vi "CANopen.vi"() -> ()   [LabVIEW 2016]
uses:
  Ctrl/CAN_Info.ctl
  Ctrl/CAN_FrameInfo.ctl
  BusStatistics/TLIBCANBusStatistics_Ctrl.ctl
  SubVIs/MessageInfo.ctl
  Ctrl/CAN_BaudInfo.ctl
  <vilib>/Platform/TimedLoop/XDataNode/timing_clust.ctl
  <vilib>/Platform/TimedLoop/XDataNode/nitl_modes.ctl
  <vilib>/Platform/TimedLoop/XDataNode/wakeup.ctl
  <vilib>/Platform/TimedLoop/XDataNode/XDataNode.xnode
  <vilib>/Platform/TimedLoop/XDataNode/XDNodeRunTimeDep.lvlib
panel:
  in  "清除总线统计":bool
  in  "使能统计功能":bool
  out "收发总数":i32
  in  "停止":bool
  in  "配置选项卡":enum32{"APP", "CAN", "DBC", "LOG"}(tab)
  in  "APP配置":T1={"应用程序名"="APP", "CAN使用通道数"=1, "LIN使用通道数"=0} {"LIN使用通道数" max=5; "CAN使用通道数" max=5}
  out "连接状态：":bool
  in  "CAN配置":T2={"硬件类型"=3, "硬件子类型"=5, "ABaudrateKbps"=500.0, "AListenOnly"=enum."Normal", "Int120Ohm"=enum."Disable", "EnableChannel"=enum."Enable", "AHwChannel"=0, "AAppChannel"=0} {"AAppChannel" items=["CHN1", "CHN2", "CHN3", "CHN4", "CHN5", "CHN6", "CHN7", "CHN8", "CHN9", "CHN10", "CHN11", "CHN12", "CHN13", "CHN14", "CHN15", "CHN16", "CHN17", "CHN18", "CHN19", "CHN20", "CHN21", "CHN22", "CHN23", "CHN24", "CHN25", "CHN26", "CHN27", "CHN28", "CHN29", "CHN30", "CHN31", "CHN32"]; "AHwChannel" items=["CHN1", "CHN2", "CHN3", "CHN4", "CHN5", "CHN6", "CHN7", "CHN8", "CHN9", "CHN10", "CHN11", "CHN12", "CHN13", "CHN14", "CHN15", "CHN16", "CHN17", "CHN18", "CHN19", "CHN20", "CHN21", "CHN22", "CHN23", "CHN24", "CHN25", "CHN26", "CHN27", "CHN28", "CHN29", "CHN30", "CHN31", "CHN32"]; "硬件子类型" items=["BUS_UNKNOWN_TYPE", "TSCAN_PRO_4", "TSCAN_LITE_2", "TSCANMini", "TSLinMini", "TSCANFDmini", "TSCAN_LIN_IO_2", "TSCAN_LITE_2", "TSCANLIN", "TSCAN_FD_Mini_1"]; "硬件类型" items=["BUS_UNKNOWN_TYPE", "TS_TCP_DEVICE", "XL_USB_DEVICE", "TS_USB_DEVICE", "PEAK_USB_DEVICE", "KVASER_USB_DEVICE", "ZLG_USB_DEVICE", "ICS_USB_DEVICE", "TS_TC1005_DEVICE"]}
  in  "StartCAN":bool
  out "CAN状态":bool
  in  "路径":path
  in  "加载dbc":bool
  in  "SupportedChannelsBased0":string
  out "out AId":u32
  in  "Blf文件路径":path=path "D:/LabviewWorkSpace/海卓项目资料/SFCV FCURig 文件夹/BottomLevel/TS_CANDrive/Test_blf/UserBlf.blf"
  in  "开启blf记录":bool
  out "TextDisplay":string
  in  "接收选项卡":enum32{"CAN", "CANopen", "DBC"}(tab)
  out "CAN数据列表":string[][](table)
  out "接收到的原始报文：":string
  out "CORecSDOData":u32 caption="接收到的数据为" format="0x%04x"
  in  "接收子索引":u8 caption="子索引" format="0x%02x"
  in  "接收索引":u16 caption="索引" format="0x%04x"
  in  "接收从站号":u8 caption="从站号" max=127
  in  "CANopenText":string
  out "当前时间":timestamp format="%<当前时间：%Y/%m/%d  %H:%M:%S>T"
  in  "消息周期":sgl=10.0
  in  "发送选项卡":enum32{"CAN", "CANopen", "DBC"}(tab)
  in  "循环周期：":u32=10 format="%d ms"
  in  "循环发送":bool
  in  "ADLC":u8=8 caption="长度：" max=64
  in  "AIsRemote":enum16{"数据帧", "远程帧"}(ring)
  in  "AIsExt":enum16{"标准帧", "扩展帧"}(ring)
  in  "AID":u32=1234 caption="ID" max=536870911 format="0x%x"
  in  "ADataArray":u8[](array[numeric])=[0, 0, 0, 0, 0, 0, 0, 0] caption="数据0x：" format="%02x"
  in  "发送通道":i32(ring) items=["CHN1", "CHN2", "CHN3", "CHN4", "CHN5", "CHN6", "CHN7", "CHN8", "CHN9", "CHN10", "CHN11", "CHN12", "CHN13", "CHN14", "CHN15", "CHN16", "CHN17", "CHN18", "CHN19", "CHN20", "CHN21", "CHN22", "CHN23", "CHN24", "CHN25", "CHN26", "CHN27", "CHN28", "CHN29", "CHN30", "CHN31", "CHN32"]
  in  "CAN发送按钮":bool
  in  "COSDOdataW":i64 caption="写入数据:" min=-32768 max=32767
  in  "写入数据类型:":T3(ring)
  out "CANopen报文预览：":string
  out "COSDOdataS":u32 caption="SDO数据" format="0x%04x"
  in  "子索引：":u8 format="0x%02x"
  in  "索引：":u16 format="0x%04x"
  in  "操作：":enum16{"SDO快速读取请求", "SDO快速写入请求"}(ring)
  in  "从站号：":u8 max=127
  in  "CANopen发送":bool
  out "tsapp_delete_cyclic_msg_can":i32
  in  "AAppChannel":i32(ring) items=["CHN1", "CHN2", "CHN3", "CHN4", "CHN5", "CHN6", "CHN7", "CHN8", "CHN9", "CHN10", "CHN11", "CHN12", "CHN13", "CHN14", "CHN15", "CHN16", "CHN17", "CHN18", "CHN19", "CHN20", "CHN21", "CHN22", "CHN23", "CHN24", "CHN25", "CHN26", "CHN27", "CHN28", "CHN29", "CHN30", "CHN31", "CHN32"]
  in  "删除周期消息":bool
  in  "周期消息":T4 {"ADLC" max=64; "AID" max=536870911}
  in  "添加周期发送消息":bool
  out "tsapp_add_cyclic_msg_can":i32
  out "接收的数据":T5[](array[typedef])
  in  "查询内容":u16(ring) items=["获取网络名称"=0, "获取dbc文件名"=1, "获取协议类型，0=CAN、1=J1939"=2, "获取信号表数量"=10, "获取CAN报文表数量"=11, "获取CANFD报文表数量"=12, "获取CANJ1939报文表数量"=13, "获取节点表数量"=14, "获取环境变量表数量"=15, "获取取值表数量"=16, "获取信号表中第idx信号所在的报文标识符"=20, "获取信号表中第idx信号值类型"=21, "获取信号表中第idx信号是否是Motorola"=22, "获取信号表中第idx信号所带的取值表在取值表列表中的索引"=23, "获取信号表中第idx信号Mux类型"=24, "获取信号表中第idx信号作为multiplexor的值"=25, "获取信号表中第idx信号在报文中的起始位"=26, "获取信号表中第idx信号的信号长度"=27, "获取信号表中第idx信号放大因子"=28, "获取信号表中第idx信号偏移量"=29, "获取信号表中第idx信号初始值"=30, "获取信号表中第idx信号最小值"=31, "获取信号表中第idx信号最大值"=32, "获取信号表中第idx信号名称"=33, "获取信号表中第idx信号单位"=34, "获取信号表中第idx信号注释"=35, "获取信号表中第idx信号所在的报文在报文表中的索引"=36, "获取信号表中第idx信号所在的报文的类型"=37, "获取信号表中第idx信号全部属性"=38, "获取CAN报文表中第idx报文类型"=40, "获取CAN报文表中第idx报文数据长度"=41, "获取CAN报文表中第idx报文标识符"=42, "获取CAN报文表中第idx报文周期"=43, "获取CAN报文表中第idx报文名称"=44, "获取CAN报文表中第idx报文注释"=45, "获取CAN报文表中第idx报文对应的发送节点的索引"=46, "获取CAN报文表中第idx报文拥有的信号数量"=47, "获取CAN报文表中第idx报文中第subidx信号在信号表中的索引"=48, "获取CAN报文表中第idx报文全部属性"=49, "获取CANFD报文表中第idx报文属性"=60, "获取CANFD报文表中第idx报文数据长度"=61, "获取CANFD报文表中第idx报文标识符"=62, "获取CANFD报文表中第idx报文周期"=63, "获取CANFD报文表中第idx报文名称"=64, "获取CANFD报文表中第idx报文注释"=65, "获取CANFD报文表中第idx报文对应的发送节点的索引"=66, "获取CANFD报文表中第idx报文拥有的信号数量"=67, "获取CANFD报文表中第idx报文中第subidx信号在信号表中的索引"=68, "获取CANFD报文表中第idx报文BRS"=69, "获取CANFD报文表中第idx报文全部属性"=70, "获取J1939报文表中第idx报文类型"=80, "获取J1939报文表中第idx报文数据长度"=81, "获取J1939报文表中第idx报文标识符"=82, "获取J1939报文表中第idx报文周期"=83, "获取J1939报文表中第idx报文名称"=84, "获取J1939报文表中第idx报文注释"=85, "获取J1939报文表中第idx报文对应的发送节点的索引"=86, "获取J1939报文表中第idx报文拥有的信号数量"=87, "获取J1939报文表中第idx报文中第subidx信号在信号表中的索引"=88, "获取CAN报文表中第idx报文全部属性"=89, "获取节点表中第idx节点地址"=100, "获取节点表中第idx节点名称"=101, "获取取值表中第idx取值表所包含的值数量"=140, "获取取值表中第idx取值表名称"=141, "获取取值表中第idx取值表中第subidx的值"=142, "获取取值表中第idx取值表全部属性"=143]
  in  "查询dbc":bool
  out "TLIBCANBusStatistics_Ctrl":T6
  out "错误输出":errorcluster
  in  "发送数据帧信息":T4={"AID"=1234, "AIsExt"=enum."STD", "AIsRemote"=enum."Data", "ADLC"=5, "ADataArray"=[0, 0, 10, 96, 8, 8]} {"ADLC" max=64; "AID" max=536870911}
  # "win32目前没有dbc属性获取，\n需要.net方式"
  # "接收"
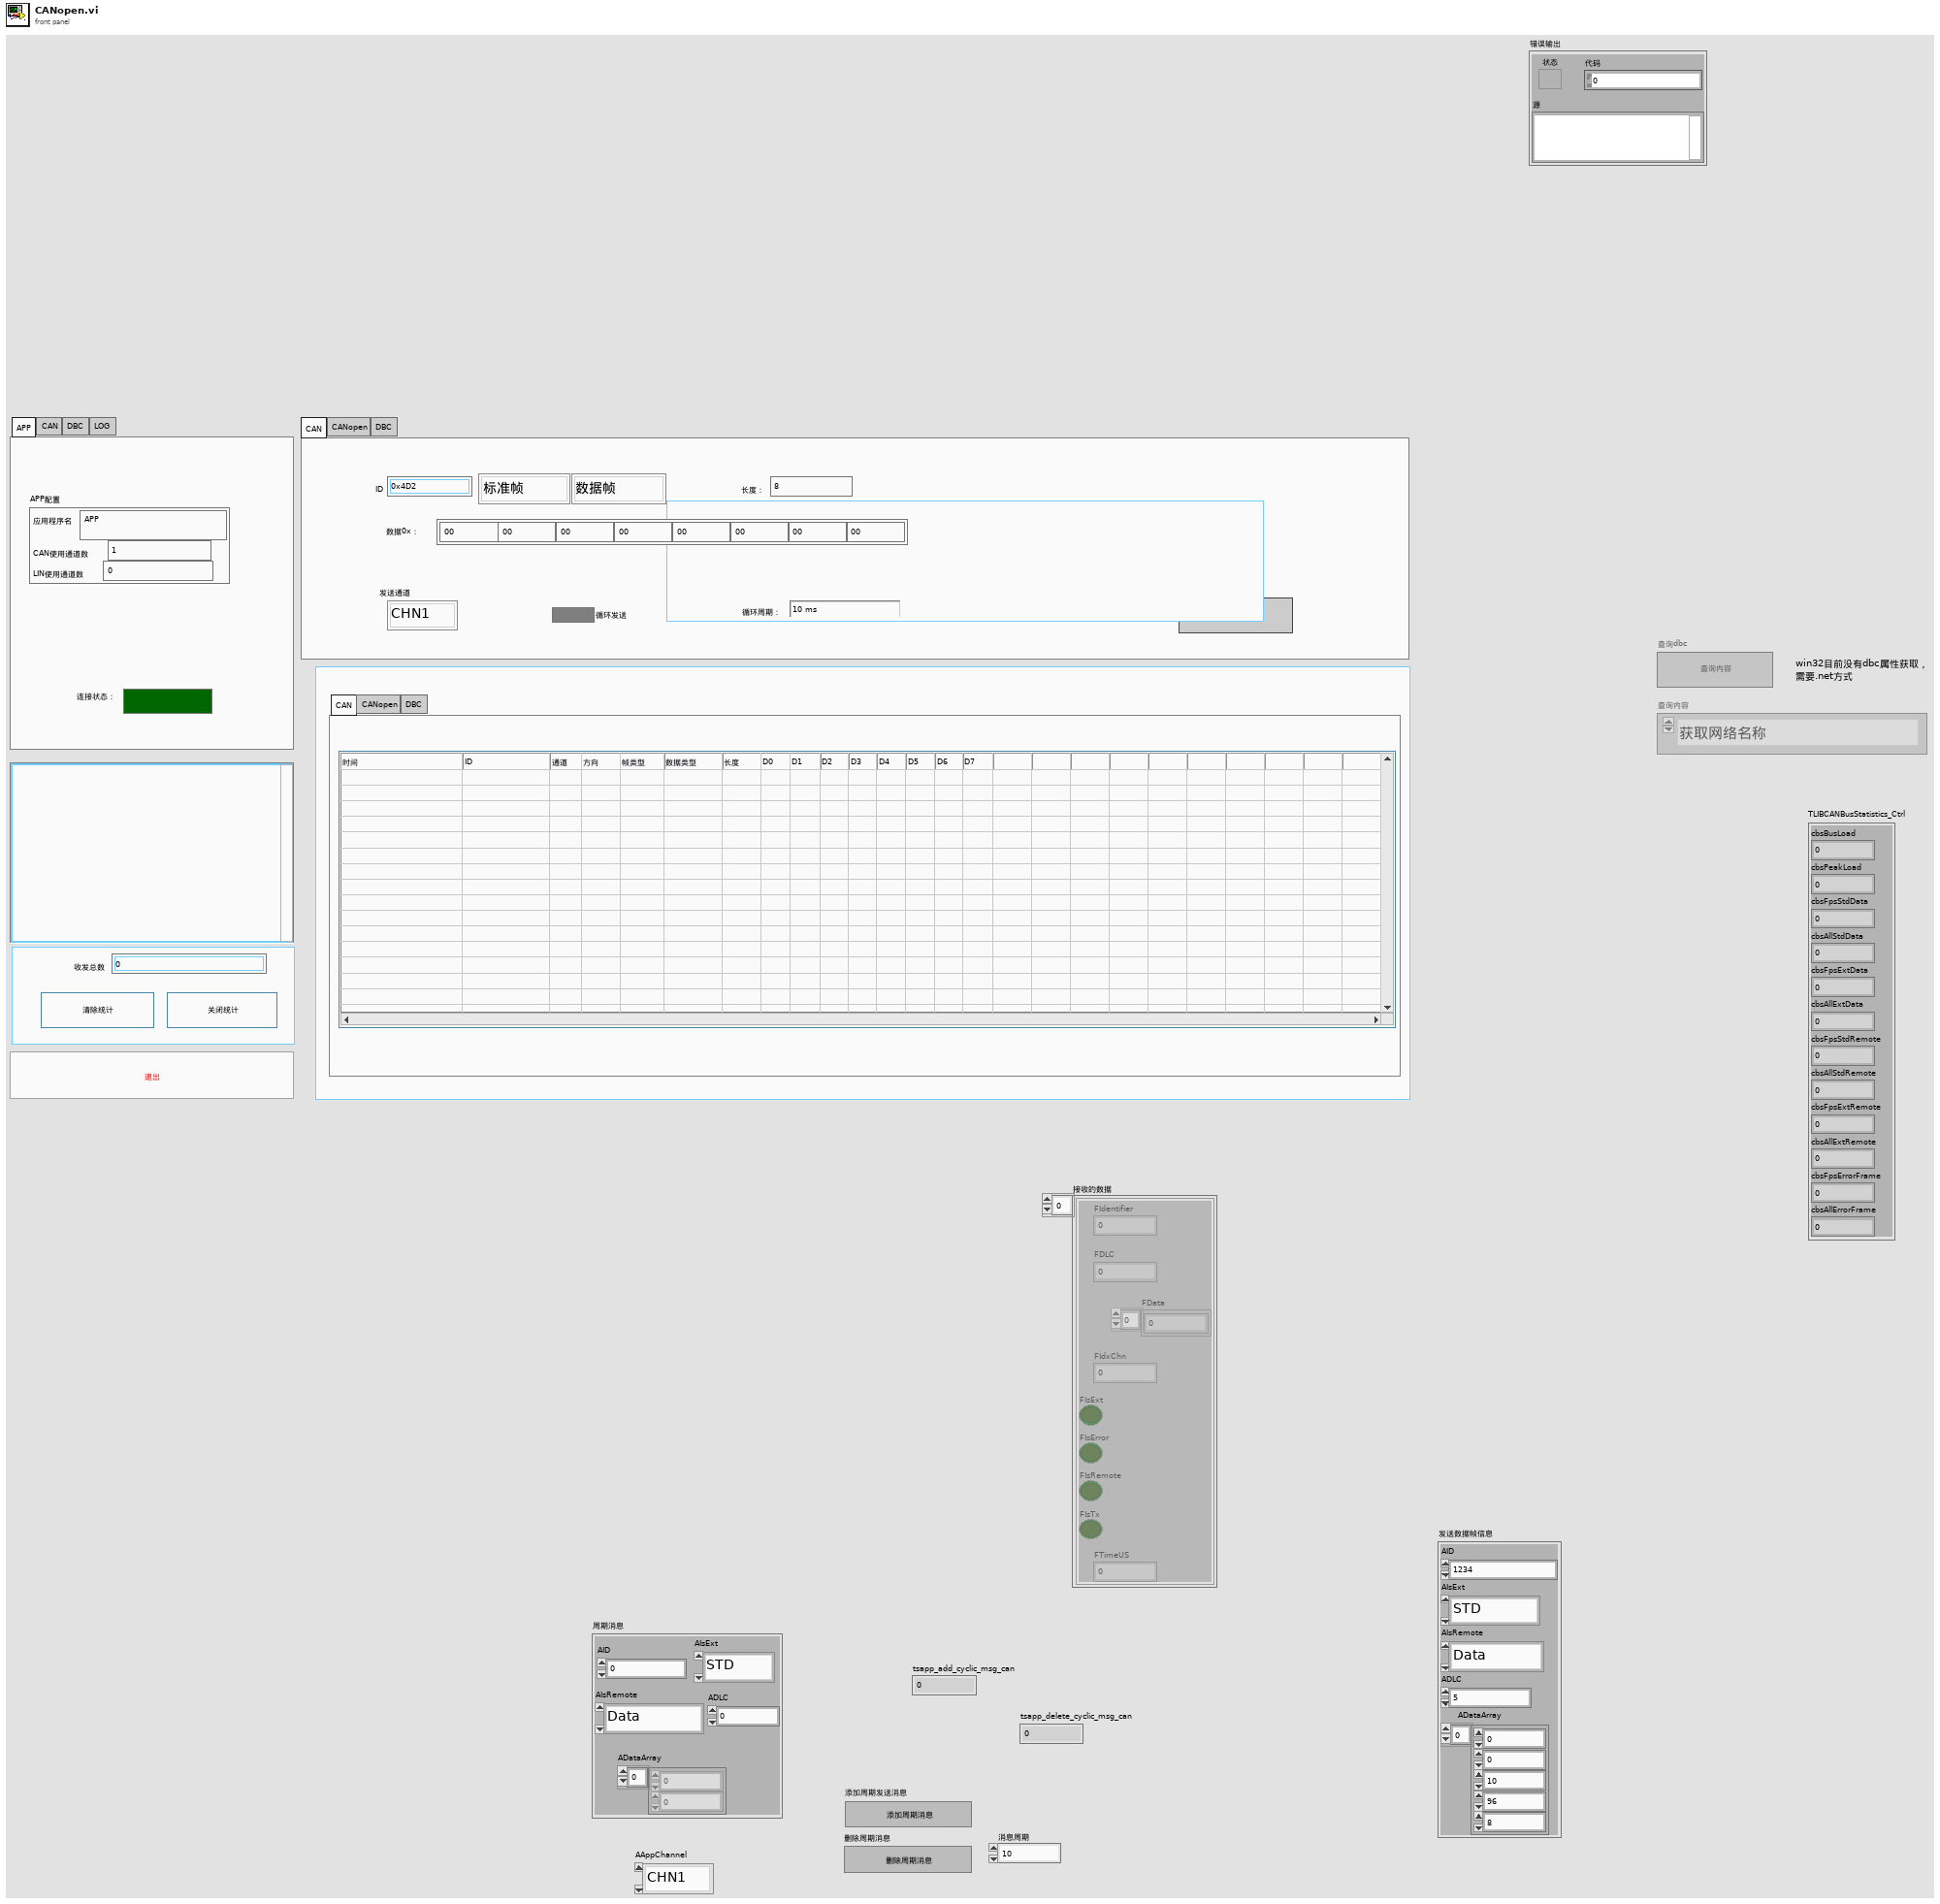
[diagram p1: front panel]
types:
  T1 = typedef "CAN_Info.ctl" = cluster{"应用程序名":string, "CAN使用通道数":u8, "LIN使用通道数":u8}
  T2 = typedef "CAN_BaudInfo.ctl" = cluster{"硬件类型":i32, "硬件子类型":i32, "ABaudrateKbps":sgl, "AListenOnly":enum16{"Normal", "ListenOnly"}, "Int120Ohm":enum16{"Disable", "Enable"}, "EnableChannel":enum16{"Disable", "Enable"}, "AHwChannel":i32, "AAppChannel":i32}
  T3 = enum16{"int8", "uint8", "int16", "uint16", "int32", "uint32"}
  T4 = typedef "CAN_FrameInfo.ctl" = cluster{"AID":u32, "AIsExt":enum16{"STD", "EXT"}, "AIsRemote":enum16{"Data", "Remote"}, "ADLC":u8, "ADataArray":u8[]}
  T5 = typedef "MessageInfo.ctl" = cluster{"FIdentifier":i32, "FDLC":u8, "FData":u8[], "FIdxChn":u8, "FIsExt":bool, "FIsError":bool, "FIsRemote":bool, "FIsTx":bool, "FTimeUS":u64}
  T6 = typedef "TLIBCANBusStatistics_Ctrl.ctl" = cluster{"cbsBusLoad":dbl, "cbsPeakLoad":dbl, "cbsFpsStdData":dbl, "cbsAllStdData":dbl, "cbsFpsExtData":dbl, "cbsAllExtData":dbl, "cbsFpsStdRemote":dbl, "cbsAllStdRemote":dbl, "cbsFpsExtRemote":dbl, "cbsAllExtRemote":dbl, "cbsFpsErrorFrame":dbl, "cbsAllErrorFrame":dbl}
  T7 = typedef "XDNodeRunTimeDep.lvlib/timing_clust.ctl" = cluster{"Expected End [f-1]":u64, "Actual End [f-1]":u64, "Finished Late? [f-1]":bool, "Expected End [i-1]":u64, "Actual End [i-1]":u64, "Finished Late? [i-1]":bool, "Expected Start [i]":u64, "Actual Start [i]":u64, "Expected Start [f]":u64, "Actual Start [f]":u64, "Source Name":string, "Structure Name":string, "Period":i64, "Deadline":i64, "Offset":i64, "Start":i64, "Priority":i32, "Timeout":i32, "Mode":T8, "Wakeup Reason":T9, "Error":errorcluster, "Source Type":string, "Secondary Source Type":string, "Global End Time":u64, "Global Start Time":u64, "Frame Duration":u64, "Iteration Duration":u64, "Assigned CPU":i32, "I/O Scan Engine Mode":u32}
  T8 = typedef "XDNodeRunTimeDep.lvlib/nitl_modes.ctl" = enum32{"No Change", "Process missed periods, maintain original phase", "Discard missed periods, maintain original phase", "Process missed periods, ignore original phase", "Discard missed periods, ignore original phase"}
  T9 = typedef "XDNodeRunTimeDep.lvlib/wakeup.ctl" = enum32{"Normal", "Aborted", "Asynchronous wakeup", "Timing source error", "Timed loop error", "Timeout"}
  T10 = enum16{"CHAN1", "CHAN2", "CHAN3", "CHAN4", "CHAN5", "CHAN6", "CHAN7", "CHAN8", "CHAN9", "CHAN10", "CHAN11", "CHAN12", "CHAN13", "CHAN14", "CHAN15", "CHAN16"}
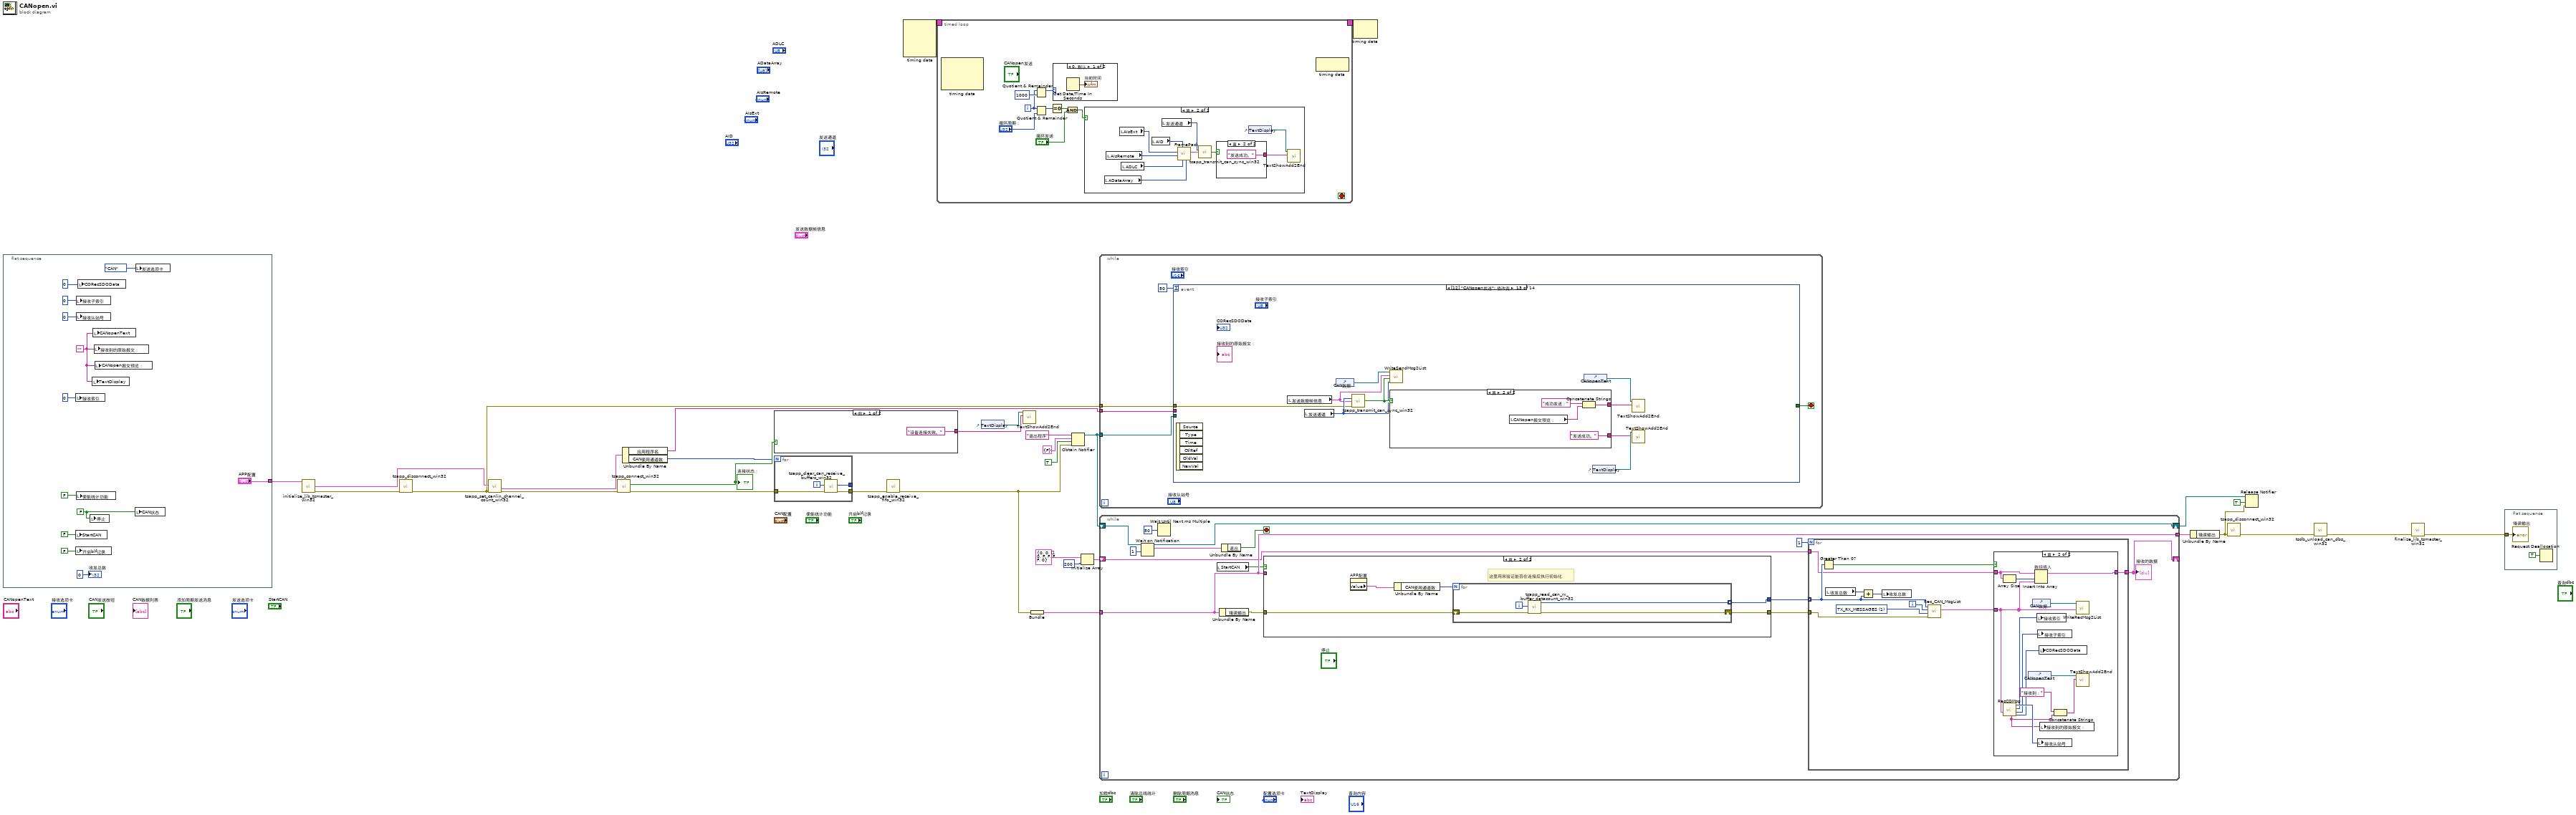
[diagram p0: block diagram]
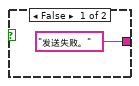
[diagram p3: hidden frame]
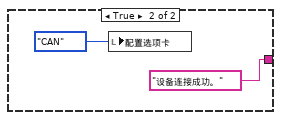
[diagram p5: hidden frame]
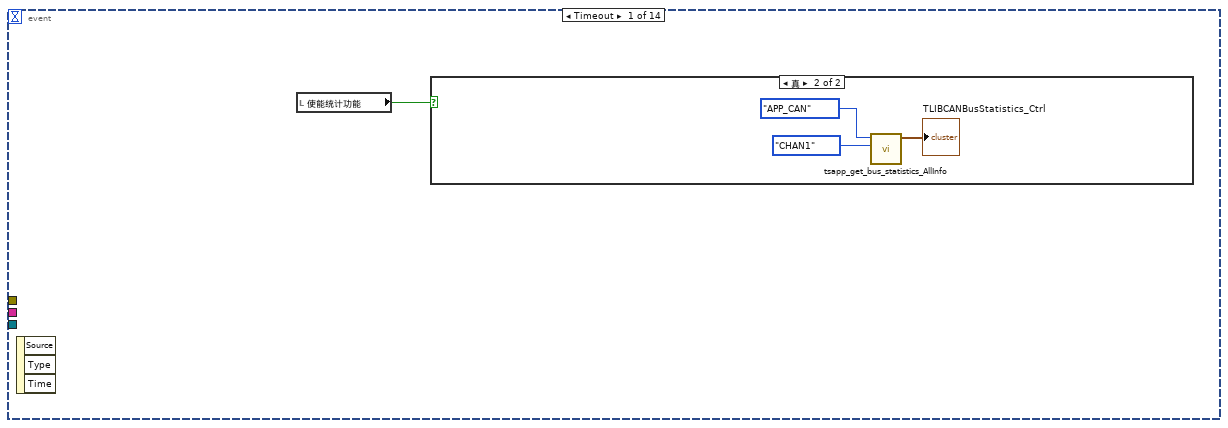
[diagram p6: hidden frame]
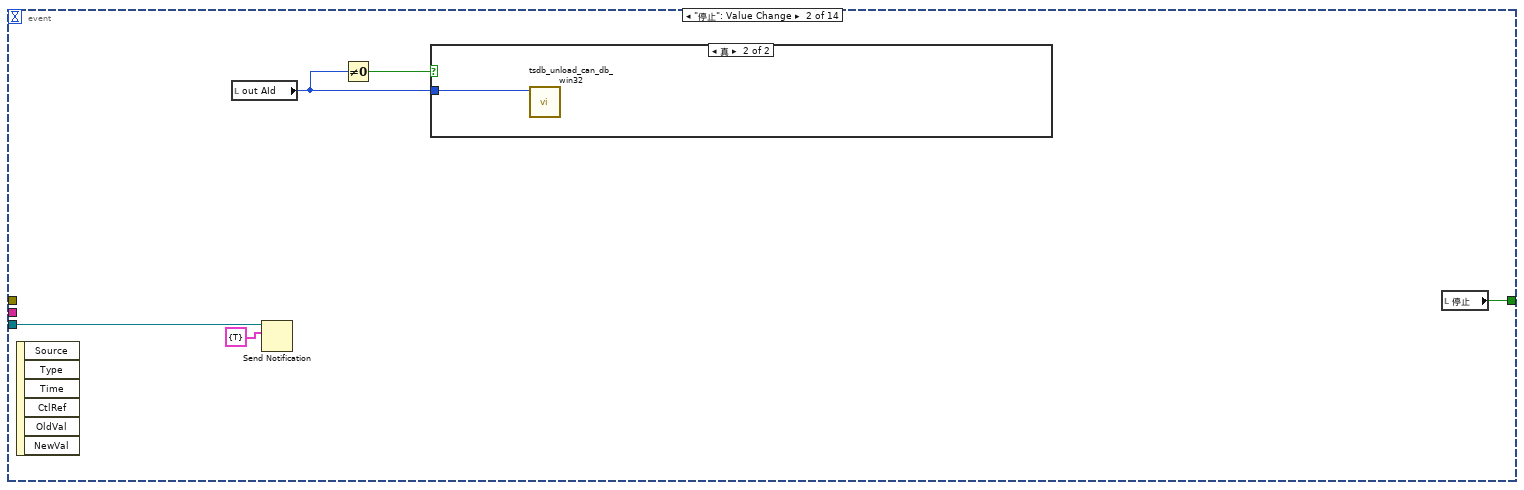
[diagram p8: hidden frame]
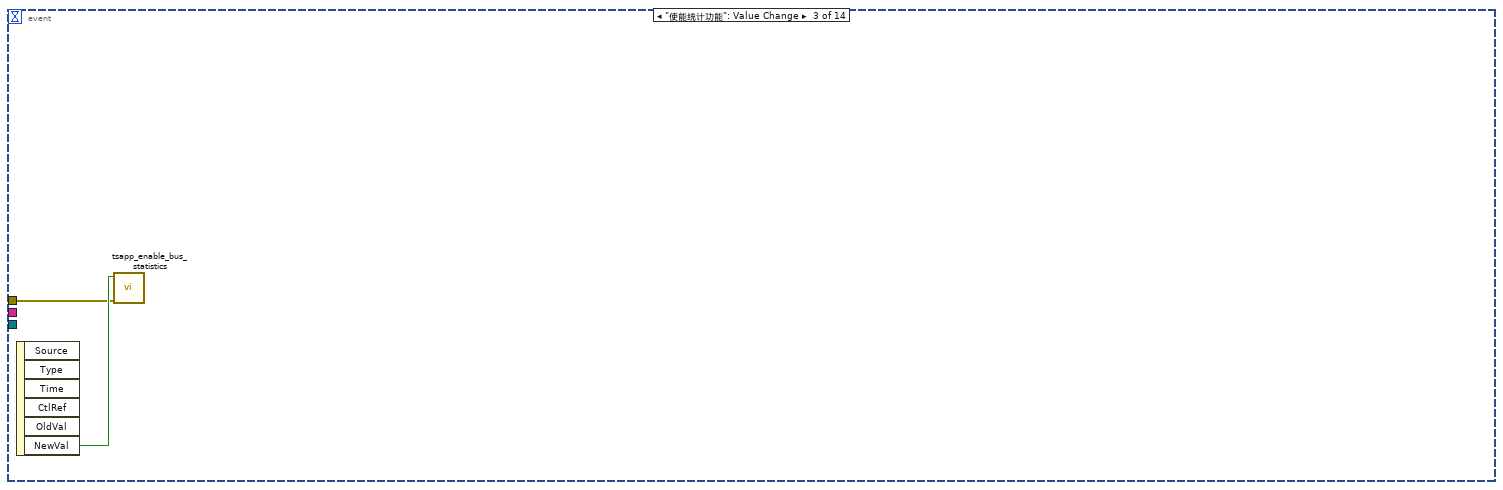
[diagram p10: hidden frame]
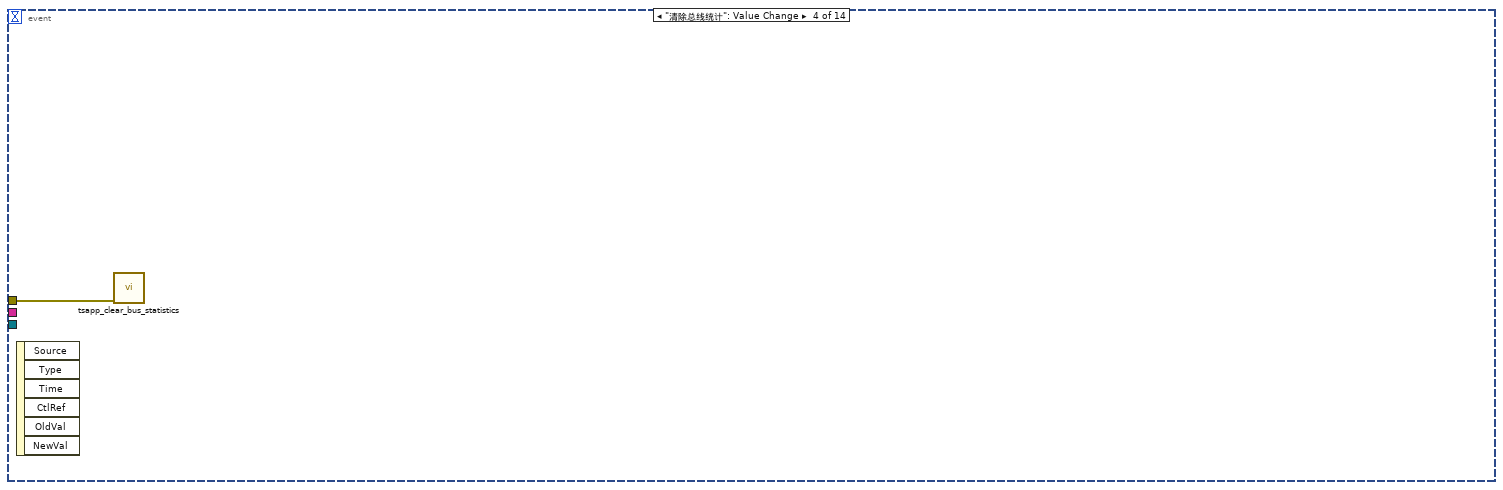
[diagram p11: hidden frame]
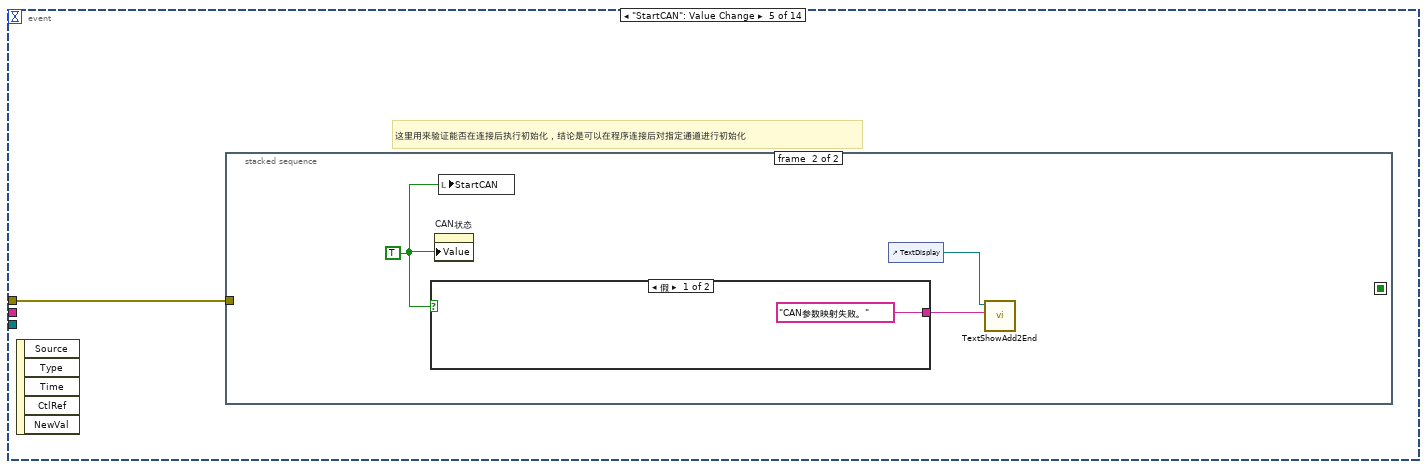
[diagram p12: hidden frame]
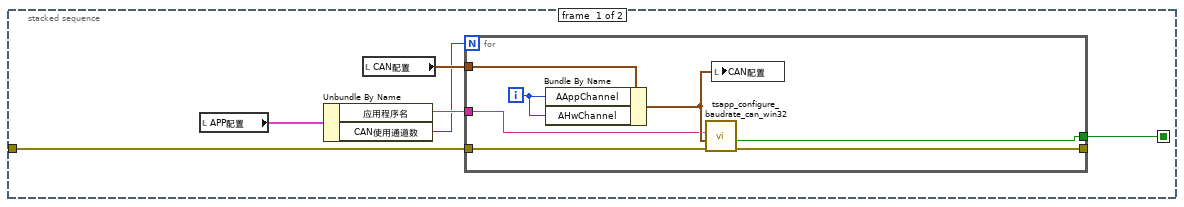
[diagram p13: hidden frame]
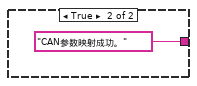
[diagram p14: hidden frame]
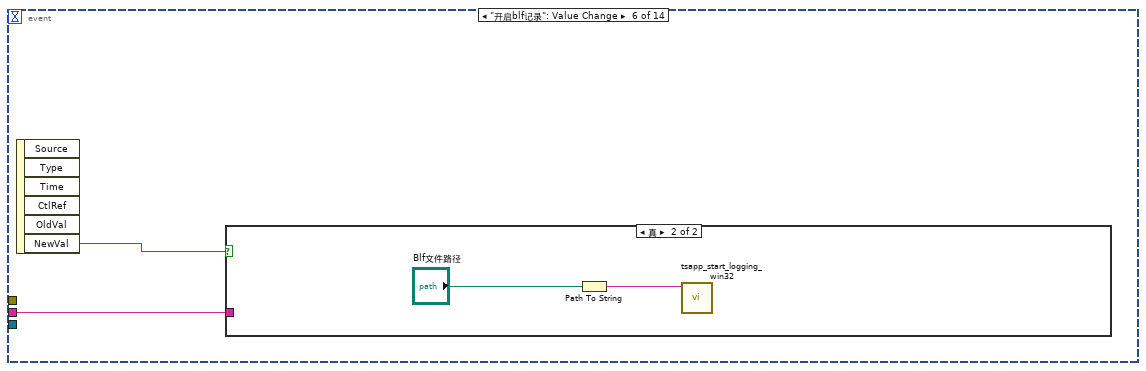
[diagram p15: hidden frame]
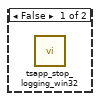
[diagram p16: hidden frame]
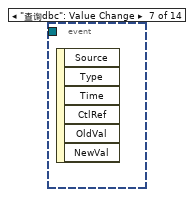
[diagram p17: hidden frame]
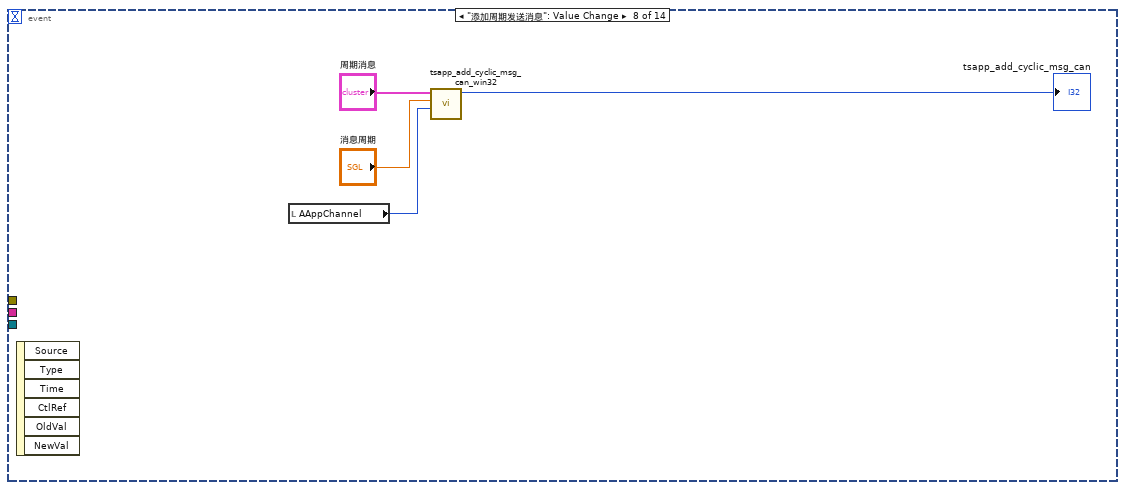
[diagram p18: hidden frame]
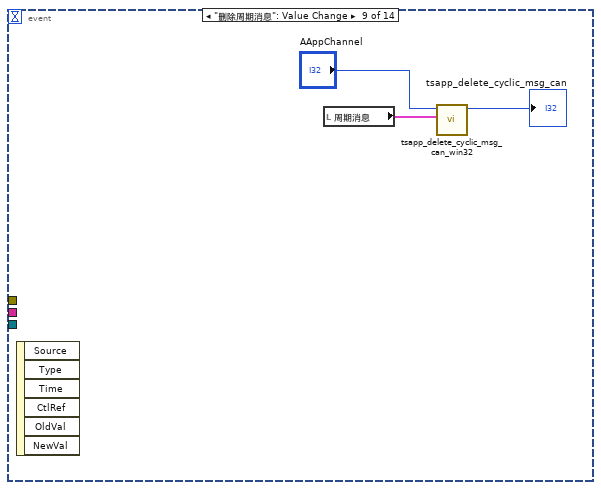
[diagram p19: hidden frame]
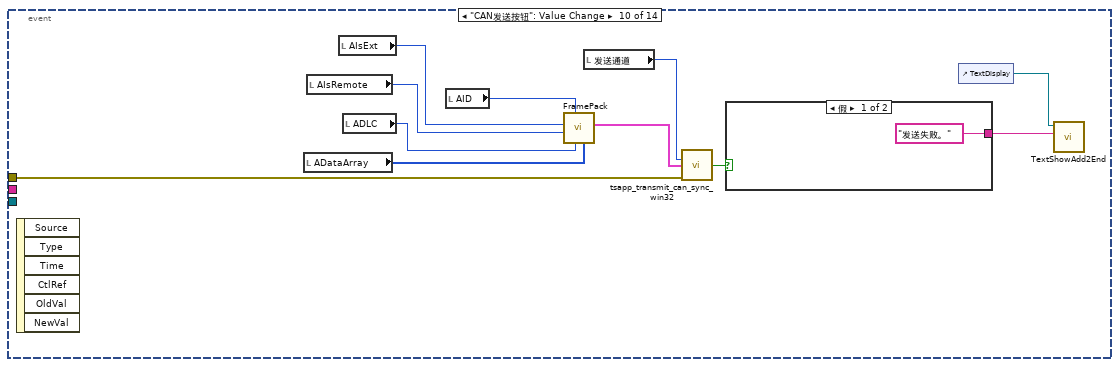
[diagram p20: hidden frame]
diagram:
  n1 = flat-sequence {
    tunnel: ["APP配置"] -> w5
    frame #0 {
      w37 = ""
      w38 = FALSE ("停止")
      n2 = local write "接收索引"(u16 0 ("接收索引")) -> ()
      n3 = local write "StartCAN"(FALSE ("初始化CAN通道")) -> ()
      n4 = local write "开启blf记录"(FALSE ("开启blf记录")) -> ()
      n5 = local write "接收子索引"(u8 0 ("接收子索引")) -> ()
      n6 = local write "接收从站号"(u8 0 ("接收从站号")) -> ()
      n7 = local write "使能统计功能"(FALSE ("使能统计功能")) -> ()
      n8 = local write "CORecSDOData"(u32 0 ("CORecSDOData")) -> ()
      n9 = local write "停止"(w38) -> ()
      n10 = local write "TextDisplay"(w37) -> ()
      n11 = local write "CANopenText"(w37) -> ()
      n12 = local write "接收到的原始报文："(w37) -> ()
      n13 = local write "CANopen报文预览："(w37) -> ()
      n14 = local write "CAN状态"(w38) -> ()
      n15 = local write "发送选项卡"(enum32{"CAN", "CANopen", "DBC"}."CAN" ("发送选项卡")) -> ()
      "收发总数" <- 0 ("接收总数")
    }
  }
  n16 = call "initialize_lib_tsmaster_win32.vi"("初始化CAN通道"=w5) -> ("InitializationInformation"=w29:T1, "错误输出"=w26:errorcluster)  [unwired: 11 in, 2 out]
  n17 = call "tsapp_disconnect_win32.vi"("错误输入（无错误）"=w26) -> ("错误输出"=w21:errorcluster)  [unwired: 8 in, 2 out]
  n18 = call "tsapp_set_canlin_channel_count_win32.vi"("错误输入（无错误）"=w21, "InitializationInformation"=w29) -> ("错误输出"=w25:errorcluster, "InitializationInformation_Out"=w9:T1)  [unwired: 7 in, 1 out]
  n19 = call "tsapp_connect_win32.vi"("错误输入（无错误）"=w25) -> ("错误输出"=w28:errorcluster, "ConnectSeccessfully"=w7:bool)  [unwired: 8 in, 1 out]
  "连接状态：" <- w7
  n20 = Unbundle By Name(w9) -> ("应用程序名"=w8:string, "CAN使用通道数"=w6:u8)
  n21 = case shown="假" w7 {
    tunnel: ["设备连接失败。" ("字符串") "设备连接成功。" ("字符串")] -> w1
    frame False {
    }
    frame True {
      n22 = local write "配置选项卡"(enum32{"APP", "CAN", "DBC", "LOG"}."CAN" ("配置选项卡")) -> ()
    }
  }
  n23 = for {
    N: w6 -> [_]
    tunnel: [w48] -> _
    tunnel: w28 -> [w50]
    tunnel: [w49] -> w27
    i -> [w47]
    n24 = call "tsapp_clear_can_receive_buffers_win32.vi"("错误输入（无错误）"=w50, "AAppChannel"=w47) -> ("错误输出"=w49:errorcluster, "tsapp_clear_can_receive_buffers"=w48:i32)  [unwired: 8 in]
  }
  n25 = call "tsapp_enable_receive_fifo_win32.vi"("错误输入（无错误）"=w27) -> ("错误输出"=w17:errorcluster)  [unwired: 10 in]
  n26 = node-c288() -> (w4:T7)  [unwired: 4 in]
  n27 = timed-loop {
    timing: w4 -> [_]
    timing-out: [_] -> w3
    i -> [w56]
    stop <- _ stop-if-true
    n28 = node-c288() -> ()  [unwired: 1 in, 4 out]
    n29 = Quotient & Remainder(x=w56, y=1000) -> (x-y*floor(x/y)=w57:i32)  [unwired: 1 out]
    n30 = Quotient & Remainder(x=w56, y="循环周期：") -> (x-y*floor(x/y)=w55:u32)  [unwired: 1 out]
    n31 = Equal To 0?(x=w55) -> (x = 0?=w53:bool)
    n32 = case shown="0, 默认" w57 {
      frame 0, Default {
        n33 = Get Date/Time In Seconds() -> (seconds since 1Jan1904=→"当前时间":timestamp)
      }
      frame 1 {
      }
    }
    n34 = And(x=w53, y="循环发送") -> (x .and. y?=w54:bool)
    n35 = case shown="真" w54 {
      frame False {
      }
      frame True {
        n36 = local read "ADataArray"() -> (w65:u8[])
        n37 = local read "AIsRemote"() -> (w63:enum16{"数据帧", "远程帧"})
        n38 = local read "AIsExt"() -> (w62:enum16{"标准帧", "扩展帧"})
        n39 = local read "ADLC"() -> (w64:u8)
        n40 = local read "AID"() -> (w61:u32)
        n41 = local read "发送通道"() -> (w68:i32)
        n42 = call "FramePack.vi"("ADataArray"=w65, "ADLC"=w64, "AID"=w61, "AIsRemote"=w63, "AIsExt"=w62) -> ("CANframe"=w66:T4)  [unwired: 6 in]
        n43 = call "tsapp_transmit_can_sync_win32.vi"("AAppChannel"=w68, "数据帧信息"=w66) -> ("TxOK?"=w67:bool)  [unwired: 11 in, 2 out]
        n44 = case shown="真" w67 {
          tunnel: ["发送失败。" ("字符串") "发送成功。" ("字符串")] -> w60
          frame False {
          }
          frame True {
          }
        }
        n45 = control-ref of="TextDisplay"() -> (w59:refnum<vi>)
        n46 = call "TextShowAdd2End.vi"("TxtAdd"=w60, "TxtBox"=w59) -> ()  [unwired: 10 in]
      }
    }
    n47 = node-c288() -> ()  [unwired: 1 in, 1 out]
  }
  n48 = control-ref of="TextDisplay"() -> (w2:refnum<vi>)
  n49 = call "TextShowAdd2End.vi"("TxtAdd"=w1, "TxtBox"=w2) -> ()  [unwired: 10 in]
  n50 = Bundle("错误输出"=w17) -> (w31:cluster{"错误输出":errorcluster})  [unwired: 1 in]
  n51 = Obtain Notifier(name (unnamed)="退出程序" ("名称（未命名）"), notification data type=cluster{"退出":bool} {"退出"=FALSE} ("退出程序"), create if not found? (T)=TRUE ("如未找到则创建？(T)"), error in (no error)=w17) -> (notifier out=w13:refnum<notifier>)  [unwired: 2 out]
  n52 = Initialize Array(T5 {"FIdentifier"=0, "FDLC"=0, "FData"=[], "FIdxChn"=0, "FIsExt"=FALSE, "FIsError"=FALSE, "FIsRemote"=FALSE, "FIsTx"=FALSE, "FTimeUS"=0} ("Receive message"), 200 ("维数大小")) -> (w10:T5[])
  n53 = while {
    tunnel: w21 -> [w78]
    tunnel: w8 -> [w75]
    tunnel: w13 -> [w74]
    stop <- w76 stop-if-true
    n54 = event shown="[12] \"CANopen发送\": 值改变" {
      selector: _ -> [_ _ _ _ _ _ _ _ _ _ _ _ _ _]
      dyn-events: _ -> [_ _ _ _ _ _ _ _ _ _ _ _ _ _]
      timeout: 50 -> [_ _ _ _ _ _ _ _ _ _ _ _ _ _]
      tunnel: w78 -> [_ _ w89 w91 w92 _ _ _ _ w132 _ _ w153 _]
      tunnel: [_ w87 _ _ _ _ _ _ _ _ _ _ _ _] -> w76
      tunnel: w75 -> [_ _ _ _ _ w111 _ _ _ _ _ _ _ _]
      tunnel: w74 -> [_ w84 _ _ _ _ _ _ _ _ _ _ _ _]
      event Timeout {
        n55 = event-data() -> ()  [unwired: 1 in, 3 out]
        n56 = local read "使能统计功能"() -> (w79:bool)
        n57 = case shown="真" w79 {
          frame False {
          }
          frame True {
            n58 = call "tsapp_get_bus_statistics_AllInfo.vi"("AIdxChn"=T10."CHAN1", "ABusType"=enum16{"APP_CAN", "APP_LIN"}."APP_CAN") -> ("TLIBCANBusStatistics_Ctrl"=→"TLIBCANBusStatistics_Ctrl":T6)  [unwired: 8 in, 1 out]
          }
        }
      }
      event "停止": Value Change {
        n59 = event-data() -> ()  [unwired: 1 in, 6 out]
        n60 = local read "out AId"() -> (w86:u32)
        n61 = Send Notification(notification=cluster{"退出":bool} {"退出"=TRUE} ("通知"), notifier=w84) -> ()  [unwired: 1 in, 2 out]
        n62 = Not Equal To 0?(x=w86) -> (x != 0?=w85:bool)
        n63 = case shown="真" w85 {
          tunnel: w86 -> [_ w88]
          frame False {
          }
          frame True {
            n64 = call "tsdb_unload_can_db_win32.vi"("out AId"=w88) -> ()  [unwired: 9 in, 2 out]
          }
        }
        n65 = local read "停止"() -> (w87:bool)
      }
      event "使能统计功能": Value Change {
        n66 = event-data() -> ("NewVal"=w90:bool)  [unwired: 1 in, 5 out]
        n67 = call "tsapp_enable_bus_statistics.vi"("错误输入（无错误）"=w89, "Enable"=w90) -> ()  [unwired: 8 in, 2 out]
      }
      event "清除总线统计": Value Change {
        n68 = event-data() -> ()  [unwired: 1 in, 6 out]
        n69 = call "tsapp_clear_bus_statistics.vi"("错误输入（无错误）"=w91) -> ()  [unwired: 9 in, 2 out]
      }
      event "StartCAN": Value Change {
        # "这里用来验证能否在连接后执行初始化，结论是可以在程序连接后对指定通道进行初始化"
        n70 = event-data() -> ()  [unwired: 1 in, 5 out]
        n71 = stacked-sequence {
          seq-local: [w93 _] -> [_ _]
          tunnel: w92 -> [w97 _]
          frame #0 {
            n72 = local read "APP配置"() -> (w96:T1)
            n73 = Unbundle By Name(w96) -> ("应用程序名"=w95:string, "CAN使用通道数"=w94:u8)
            n74 = local read "CAN配置"() -> (w98:T2)
            n75 = for {
              N: w94 -> [_]
              tunnel: [w104] -> w93
              tunnel: w97 -> [w105]
              tunnel: [w103] -> _
              tunnel: w98 -> [w102]
              tunnel: w95 -> [w99]
              i -> [w101]
              n76 = Bundle By Name(cluster=w102, "AAppChannel"=w101, "AHwChannel"=w101) -> (w100:T2)
              n77 = call "tsapp_configure_baudrate_can_win32.vi"("AppName"=w99, "配置波特率"=w100, "错误输入（无错误）"=w105) -> ("InitSts"=w104:bool, "错误输出"=w103:errorcluster)  [unwired: 6 in]
              n78 = local write "CAN配置"(w100) -> ()
            }
          }
          frame #1 {
            w108 = TRUE ("初始化CAN通道")
            n79 = case shown="假" w108 {
              tunnel: ["CAN参数映射失败。" ("字符串") "CAN参数映射成功。" ("字符串")] -> w106
              frame False {
              }
              frame True {
              }
            }
            n80 = property on="CAN状态" class="Bool (严格)"("Value"=w108) -> ()  [unwired: 2 in, 2 out]
            n81 = local write "StartCAN"(w108) -> ()
            n82 = control-ref of="TextDisplay"() -> (w107:refnum<vi>)
            n83 = call "TextShowAdd2End.vi"("TxtAdd"=w106, "TxtBox"=w107) -> ()  [unwired: 10 in]
          }
        }
      }
      event "开启blf记录": Value Change {
        n84 = event-data() -> ("NewVal"=w112:bool)  [unwired: 1 in, 5 out]
        n85 = case shown="真" w112 {
          tunnel: w111 -> [_ _]
          frame False {
            n86 = call "tsapp_stop_logging_win32.vi"() -> ()  [unwired: 10 in, 2 out]
          }
          frame True {
            n87 = Path To String(path="Blf文件路径") -> (string=w113:string)
            n88 = call "tsapp_start_logging_win32.vi"("AFileName"=w113) -> ()  [unwired: 9 in, 2 out]
          }
        }
      }
      event "查询dbc": Value Change {
        n89 = event-data() -> ()  [unwired: 1 in, 6 out]
      }
      event "添加周期发送消息": Value Change {
        n90 = event-data() -> ()  [unwired: 1 in, 6 out]
        n91 = local read "AAppChannel"() -> (w115:i32)
        n92 = call "tsapp_add_cyclic_msg_can_win32.vi"("AAppChannel"=w115, "APeriodMS"="消息周期", "数据帧信息"="周期消息") -> ("tsapp_add_cyclic_msg_can"=→"tsapp_add_cyclic_msg_can":i32)  [unwired: 7 in, 1 out]
      }
      event "删除周期消息": Value Change {
        n93 = event-data() -> ()  [unwired: 1 in, 6 out]
        n94 = local read "周期消息"() -> (w119:T4)
        n95 = call "tsapp_delete_cyclic_msg_can_win32.vi"("数据帧信息"=w119, "AAppChannel"="AAppChannel") -> ("tsapp_delete_cyclic_msg_can"=→"tsapp_delete_cyclic_msg_can":i32)  [unwired: 8 in, 1 out]
      }
      event "CAN发送按钮": Value Change {
        n96 = event-data() -> ()  [unwired: 1 in, 6 out]
        n97 = local read "ADataArray"() -> (w127:u8[])
        n98 = local read "AIsRemote"() -> (w129:enum16{"数据帧", "远程帧"})
        n99 = local read "AIsExt"() -> (w130:enum16{"标准帧", "扩展帧"})
        n100 = local read "ADLC"() -> (w128:u8)
        n101 = local read "AID"() -> (w131:u32)
        n102 = call "FramePack.vi"("ADataArray"=w127, "ADLC"=w128, "AID"=w131, "AIsRemote"=w129, "AIsExt"=w130) -> ("CANframe"=w126:T4)  [unwired: 6 in]
        n103 = local read "发送通道"() -> (w124:i32)
        n104 = call "tsapp_transmit_can_sync_win32.vi"("AAppChannel"=w124, "数据帧信息"=w126, "错误输入（无错误）"=w132) -> ("TxOK?"=w125:bool)  [unwired: 10 in, 2 out]
        n105 = case shown="假" w125 {
          tunnel: ["发送失败。" ("字符串") "发送成功。" ("字符串")] -> w123
          frame False {
          }
          frame True {
          }
        }
        n106 = control-ref of="TextDisplay"() -> (w122:refnum<vi>)
        n107 = call "TextShowAdd2End.vi"("TxtAdd"=w123, "TxtBox"=w122) -> ()  [unwired: 10 in]
      }
      event "发送选项卡": Value Change {
        n108 = event-data() -> ("NewVal"=w135:enum32{"CAN", "CANopen", "DBC"})  [unwired: 1 in, 5 out]
        n109 = case shown="\"CANopen\"" w135 {
          frame "CAN", Default {
          }
          frame "CANopen" {
            n110 = local write "循环发送"(FALSE ("循环发送")) -> ()
            n111 = local write "接收选项卡"(enum32{"CAN", "CANopen", "DBC"}."CANopen" ("接收选项卡")) -> ()
          }
          frame "DBC" {
          }
        }
      }
      event "CANopen报文预览：", "COSDOdataW", "子索引：", "索引：", "操作：", "从站号：", "写入数据类型:": Value Change {
        n112 = event-data() -> ()  [unwired: 1 in, 6 out]
        n113 = control-ref of="COSDOdataW"() -> (w139:refnum<vi>)
        n114 = control-ref of="COSDOdataS"() -> (w138:refnum<vi>)
        n115 = control-ref of="写入数据类型:"() -> (w142:refnum<vi>)
        n116 = call "CanopenSendMsgPack.vi"("COSDOdataW"=w139, "写入数据类型"=w142, "操作："="操作：", "COSDOdataS"=w138, "从站号："="从站号：", "索引："="索引：", "子索引："="子索引：") -> ("发送数据帧信息输出"=w146:T4, "字符串"=→"CANopen报文预览：":string)  [unwired: 7 in]
        n117 = local write "发送数据帧信息"(w146) -> ()
      }
      event "CANopen发送": Value Change {
        n118 = event-data() -> ()  [unwired: 1 in, 6 out]
        n119 = local read "发送数据帧信息"() -> (w151:T4)
        n120 = local read "发送通道"() -> (w154:i32)
        n121 = control-ref of="CAN数据列表"() -> (w152:refnum<vi>)
        n122 = call "tsapp_transmit_can_sync_win32.vi"("AAppChannel"=w154, "数据帧信息"=w151, "错误输入（无错误）"=w153) -> ("TxOK?"=w155:bool)  [unwired: 10 in, 2 out]
        n123 = call "WriteSendMsg2List.vi"("发送通道"=w154, "SendOK"=w155, "CANframe"=w151, "Table输入"=w152) -> ()  [unwired: 8 in]
        n124 = case shown="真" w155 {
          tunnel: [w156 "发送成功。" ("字符串")] -> w149
          tunnel: [w156 w159] -> w148
          frame False {
            w156 = "发送失败。" ("字符串")
          }
          frame True {
            n125 = local read "CANopen报文预览："() -> (w160:string)
            n126 = Concatenate Strings("成功发送：" ("字符串"), w160) -> (w159:string)
          }
        }
        n127 = control-ref of="CANopenText"() -> (w147:refnum<vi>)
        n128 = control-ref of="TextDisplay"() -> (w150:refnum<vi>)
        n129 = call "TextShowAdd2End.vi"("TxtAdd"=w148, "TxtBox"=w147) -> ()  [unwired: 10 in]
        n130 = call "TextShowAdd2End.vi"("TxtAdd"=w149, "TxtBox"=w150) -> ()  [unwired: 10 in]
      }
      event "加载dbc": Value Change {
        n131 = event-data() -> ()  [unwired: 1 in, 5 out]
        n132 = Not Equal?(x=path "", y="路径") -> (x != y?=w162:bool)
        n133 = case shown="真" w162 {
          tunnel: "路径" -> [_ w165]
          frame False {
          }
          frame True {
            n134 = call "tsdb_load_can_db_win32.vi"("ASupportedChannelsBased0"="SupportedChannelsBased0", "路径"=w165) -> ("out AId"=→"out AId":u32)  [unwired: 7 in, 2 out]
          }
        }
      }
    }
  }
  n135 = while {
    tunnel: w31 -> [w180]
    tunnel: [w180] -> w30
    shift-right: [w167] -> _
    shift-left: w10 -> [w178]
    shift-right: [w170] -> w16
    shift-left: w13 -> [w172]
    stop <- w168 stop-if-true
    n136 = Wait on Notification(notifier=w172, timeout in ms (-1)=1 ("超时毫秒(-1)")) -> (notifier out=w170:refnum<notifier>, notification=w169:cluster{"退出":bool})  [unwired: 2 in, 2 out]
    n137 = Wait Until Next ms Multiple(millisecond multiple=u32 50 ("毫秒倍数")) -> ()  [unwired: 1 out]
    n138 = local read "StartCAN"() -> (w176:bool)
    n139 = Unbundle By Name(w180) -> ("错误输出"=w175:errorcluster)
    n140 = Unbundle By Name(w169) -> ("退出"=w168:bool)
    n141 = case shown="真" w176 {
      tunnel: w180 -> [_ _]
      tunnel: [w206 w211] -> w179
      tunnel: [i32[] [] w210] -> w177
      tunnel: w175 -> [w206 w209]
      frame False {
      }
      frame True {
        # "这里用来验证能否在连接后执行初始化"
        n142 = property on="APP配置" class="Clust (严格)"() -> ("Value"=w208:T1)  [unwired: 2 in, 2 out]
        n143 = Unbundle By Name(w208) -> ("CAN使用通道数"=w207:u8)
        n144 = for {
          N: w207 -> [_]
          tunnel: [w214] -> w210 mode=indexing
          shift-right: [w215] -> w211
          shift-left: w209 -> [w213]
          i -> [w212]
          n145 = call "tsapp_read_can_rx_buffer_datacount_win32.vi"("错误输入（无错误）"=w213, "AAppChannel"=w212) -> ("错误输出"=w215:errorcluster, "tsapp_read_can_buffer_datacount"=w214:i32)  [unwired: 7 in, 1 out]
        }
      }
    }
    n146 = for {
      N: 1 -> [_]
      tunnel: w179 -> [w190]
      tunnel: w177 -> [w188] mode=indexing
      tunnel: w178 -> [w182]
      tunnel: [w181] -> w167
      i -> [w189]
      w184 = u8 1 items=["ONLY_RX_MESSAGES", "TX_RX_MESSAGES"] ("AOnlyRx")
      n147 = Greater Than 0?(x=w188) -> (x > 0?=w183:bool)
      n148 = local read "收发总数"() -> (w187:i32)
      n149 = Add(x=w187, y=w188) -> (x+y=w186:i32)
      n150 = local write "收发总数"(w186) -> ()
      n151 = call "Rec_CAN_MsgList.vi"("错误输入（无错误）"=w190, "AOnlyRx"=w184, "AAppChannel输入"=w189, "ACANBufferSize"=w188) -> ("tsapp_receive_can_messageList"=w185:T5[])  [unwired: 5 in, 2 out]
      n152 = case shown="真" w183 {
        tunnel: w185 -> [_ w201]
        tunnel: w182 -> [w191 w204]
        tunnel: [w191 w202] -> w181
        frame False {
        }
        frame True {
          n153 = Array Size(array=w204) -> (size(s)=w203:i32)
          n154 = call "RecCOMsg.vi"("tsapp_receive_can_messageList"=w201) -> ("CORecSDOData"=w197:u32, "接收子索引"=w198:u8, "接收索引"=w199:u16, "接收从站号"=w200:u8, "接收到的原始报文："=w195:string)  [unwired: 6 in]
          n155 = control-ref of="CANopenText"() -> (w193:refnum<vi>)
          n156 = control-ref of="CAN数据列表"() -> (w194:refnum<vi>)
          n157 = Insert Into Array "数组插入"(array=w204, index=w203, new element=w201) -> (w202:T5[])
          n158 = local write "接收索引"(w199) -> ()
          n159 = local write "接收子索引"(w198) -> ()
          n160 = local write "接收从站号"(w200) -> ()
          n161 = local write "CORecSDOData"(w197) -> ()
          n162 = local write "接收到的原始报文："(w195) -> ()
          n163 = Concatenate Strings("接收到：", w195) -> (w192:string)
          n164 = call "WriteRecMsg2List.vi"("tsapp_receive_can_messageList"=w201, "Table输入"=w194) -> ()  [unwired: 10 in]
          n165 = call "TextShowAdd2End.vi"("TxtAdd"=w192, "TxtBox"=w193) -> ()  [unwired: 10 in]
        }
      }
    }
    "接收的数据" <- w167
  }
  n166 = node-c288(w3) -> ()  [unwired: 1 out]
  n167 = Unbundle By Name(w30) -> ("错误输出"=w14:errorcluster)
  n168 = call "tsapp_disconnect_win32.vi"("错误输入（无错误）"=w14) -> ("错误输出"=w23:errorcluster)  [unwired: 8 in, 2 out]
  n169 = Release Notifier(notifier=w16, force destroy? (F)=TRUE ("强制销毁？(F)"), error in (no error)=w14) -> ()  [unwired: 3 out]
  n170 = call "tsdb_unload_can_dbs_win32.vi"("错误输入（无错误）"=w23) -> ("错误输出"=w22:errorcluster)  [unwired: 9 in, 1 out]
  n171 = call "finalize_lib_tsmaster_win32.vi"("错误输入（无错误）"=w22) -> ("错误输出"=w24:errorcluster)  [unwired: 10 in]
  n172 = flat-sequence {
    tunnel: w24 -> [w217]
    frame #0 {
      n173 = Request Deallocation(TRUE ("标志")) -> ()
      "错误输出" <- w217
    }
  }
